vi "project.vi"() -> ()   [LabVIEW 2021]
panel:
  in  "System Mode: Automatic":bool
  in  "Passcode":string
  out "Air Conditioning 2":dbl
  out "Lighting Level 2":u8(slide) scale=0.0..100.0
  out "Home Theater 2":bool
  in  "Time of the Day":timestamp
  in  "Atmospheric Temperature":dbl(slide) scale=0.0..100.0
  out "Air Conditioning":dbl
  out "Lighting Level":u8(slide) scale=0.0..100.0
  out "Home Theater":bool
  # "Living Room"
  # "deg C"
  # "BR1: Master"
  # "deg C"
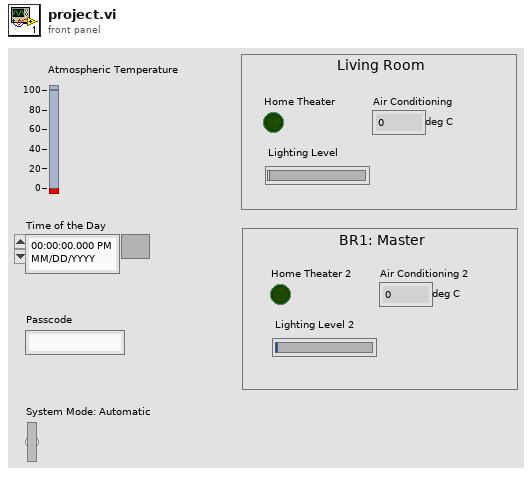
[diagram p1: front panel]
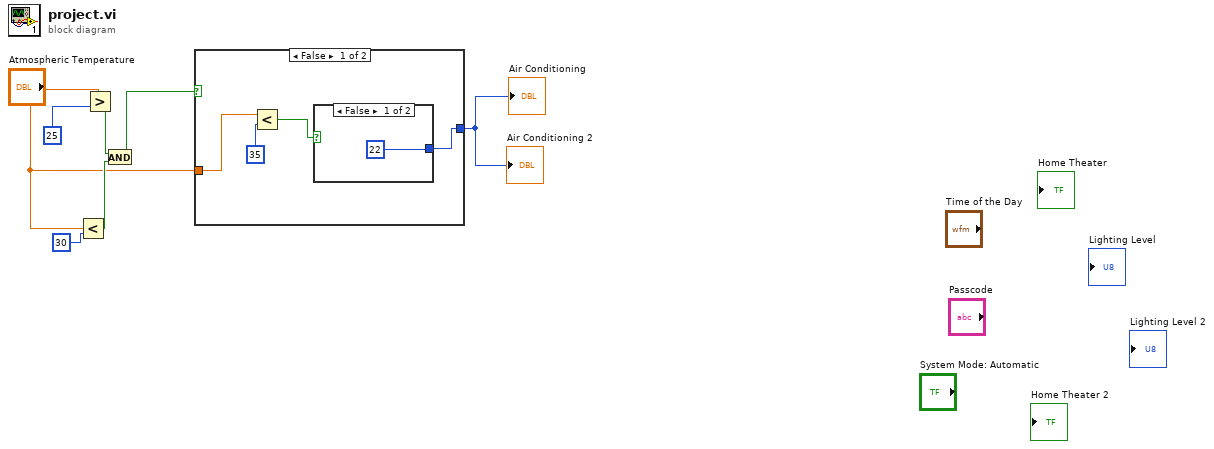
[diagram p0: block diagram]
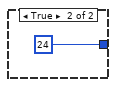
[diagram p2: hidden frame]
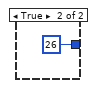
[diagram p3: hidden frame]
diagram:
  n1 = Less?(x="Atmospheric Temperature", y=30) -> (x < y?=w4:bool)
  n2 = Greater?(x="Atmospheric Temperature", y=25) -> (0:w5:bool)
  n3 = And(x=w5, y=w4) -> (x .and. y?=w3:bool)
  n4 = case shown="False" w3 {
    tunnel: [w8 26] -> w1
    tunnel: "Atmospheric Temperature" -> [w11 _]
    frame False {
      n5 = Less?(x=w11, y=35) -> (x < y?=w9:bool)
      n6 = case shown="False" w9 {
        tunnel: [22 24] -> w8
        frame False {
        }
        frame True {
        }
      }
    }
    frame True {
    }
  }
  "Air Conditioning" <- w1
  "Air Conditioning 2" <- w1
